vi "test_basic_init.vi"() -> (3 "test_result":T1)   [LabVIEW 2015]
uses:
  tester_result.ctl
  input/input.lvclass
  output/Output.lvclass
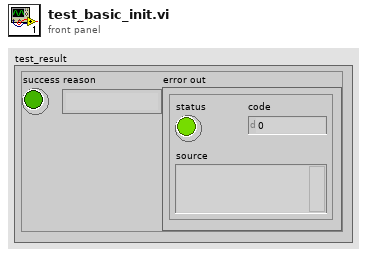
[diagram p1: front panel]
types:
  T1 = typedef "tester_result.ctl" = cluster{"success":bool, "reason":string, "error out":errorcluster}
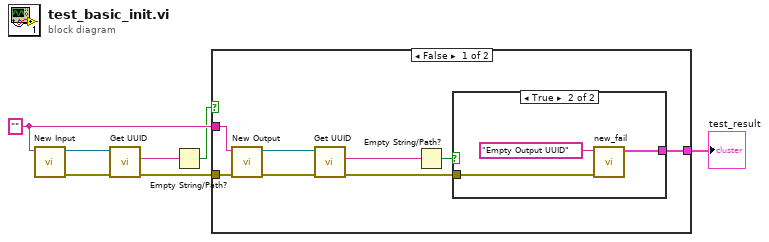
[diagram p0: block diagram]
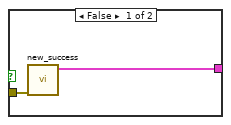
[diagram p2: hidden frame]
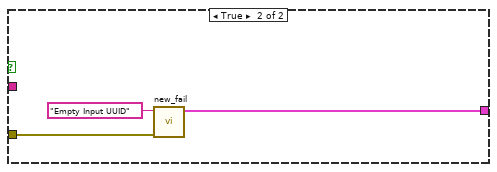
[diagram p3: hidden frame]
diagram:
  w7 = "" ("Descriptor")
  n1 = call "New Input.vi"("Descriptor"=w7) -> ("error out"=w5:errorcluster, "input out"=w4:refnum<class "input.lvclass">)  [unwired: 9 in]
  n2 = call "Get UUID.vi"("error in (no error)"=w5, "input in"=w4) -> ("error out"=w3:errorcluster, "UUID"=w2:string)  [unwired: 7 in, 1 out]
  n3 = Empty String/Path?(string/path=w2) -> (empty?=w1:bool)
  n4 = case shown="False" w1 {
    tunnel: w7 -> [w15 _]
    tunnel: [w14 w21] -> w6
    tunnel: w3 -> [w13 w22]
    frame False {
      n5 = call "New Output.vi"("error in (no error)"=w13, "Descriptor"=w15) -> ("error out"=w12:errorcluster, "output"=w11:refnum<class "Output.lvclass">)  [unwired: 8 in]
      n6 = call "Get UUID.vi"("error in (no error)"=w12, "Output in"=w11) -> ("error out"=w10:errorcluster, "UUID"=w9:string)  [unwired: 7 in, 1 out]
      n7 = Empty String/Path?(string/path=w9) -> (empty?=w8:bool)
      n8 = case shown="True" w8 {
        tunnel: [w17 w19] -> w14
        tunnel: w10 -> [w16 w18]
        frame False {
          n9 = call "new_success.vi"("error out"=w16) -> ("result"=w17:T1)  [unwired: 10 in]
        }
        frame True {
          n10 = call "new_fail.vi"("error out"=w18, "reason"="Empty Output UUID") -> ("result"=w19:T1)  [unwired: 9 in]
        }
      }
    }
    frame True {
      n11 = call "new_fail.vi"("error out"=w22, "reason"="Empty Input UUID") -> ("result"=w21:T1)  [unwired: 9 in]
    }
  }
  "test_result" <- w6
